vi "S2C_M2p5942_Poly_Acquisition.vi"(8 "Error In":errorcluster, 10 "Acquisition":T1={"Single Shot"=FALSE, "Loop"=FALSE, "Force Trigger"=FALSE, "Status"="<Status>", "Stop"=FALSE, "Graph"=[]}, 11 "Settings":T2={"Driver"="M2p5942", "Command"="Acquisition", "Return"="ErrorStatus", "Parameters"="", "Timeout"=10.0}) -> (0 "Error Out":errorcluster, 3 "Response":string)   [LabVIEW 2015]
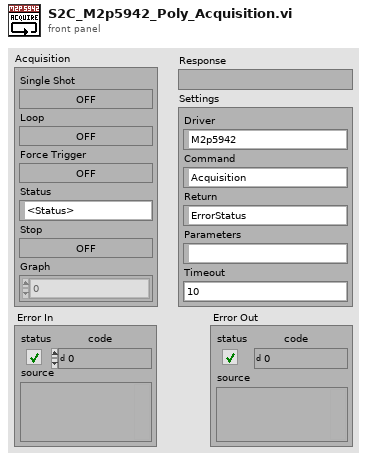
[diagram p1: front panel]
types:
  T1 = cluster{"Single Shot":bool, "Loop":bool, "Force Trigger":bool, "Status":string, "Stop":bool, "Graph":sgl[][]}
  T2 = cluster{"Driver":string, "Command":string, "Return":string, "Parameters":string, "Timeout":dbl}
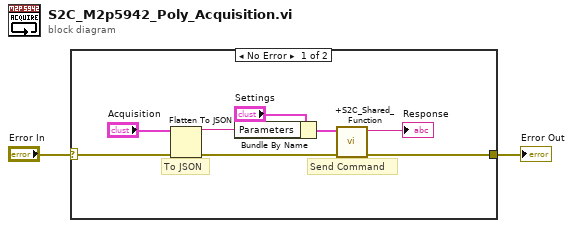
[diagram p0: block diagram]
diagram:
  n1 = case shown="No Error" "Error In" {
    selector: "Error In" -> [w6 w11]
    tunnel: [w5 w11] -> w1
    frame No Error {
      # "To JSON"
      # "Send Command"
      n2 = Flatten To JSON(anything="Acquisition", error in (no error)=w6) -> (JSON string=w7:string, 11:w9:errorcluster)  [unwired: 1 in]
      n3 = Bundle By Name(cluster="Settings", "Parameters"=w7) -> (w10:T2)
      n4 = call "+S2C_Shared_Function.vi"("Error In"=w9, "Settings"=w10) -> ("Error Out"=w5:errorcluster, "Response"=→"Response":string)  [unwired: 8 in]
    }
    frame Error {
    }
  }
  "Error Out" <- w1
